vi "test All Verifies With Labels.vi"(8 "error in":errorcluster, 11 "Testing Approval Tests in":refnum<class "VITester Extension Tests.lvclass">) -> (0 "error out":errorcluster, 3 "Testing Approval Tests in":refnum<class "VITester Extension Tests.lvclass">)   [LabVIEW 2025, in "VITester Extension Tests.lvclass"]
uses:
  VITester Extension Tests.lvclass
  C:/Program Files/National Instruments/LabVIEW 2026/vi.lib/Addons/_JKI Toolkits/VI Tester/TestCase.llb/TestCase.lvclass
  Source/Approval Tests/Options/Options.lvclass/Options.ctl
  Source/Approval Tests/Naming Data/Naming Data.lvclass/Naming Data.ctl
  Caraya.Tests/Caraya Extension Tests/Utility Greet.vi
  Source/Approval Tests/Options/Options.lvclass
  Source/Approval Tests/Scrubber/Scrubber.lvclass
  Source/Approval Tests/Namer/Namer.lvclass
  Source/Approval Tests/Naming Data/Naming Data.lvclass
  Source/Approval Tests/Reporter/Reporter.lvclass
  Source/Approval Tests/Text Comparator/Text Comparator.lvclass
  VITester Extension Tests.lvclass/VITester Extension Tests.ctl
  24d0000c-8485-4d5f-9e8a-c81d323cd4a2.vi
  25835d91-223e-4457-8654-ed94975679ce.vi
  Caraya.Tests/Caraya Extension Tests/Caraya Extension Tests.lvclass
  1e735b7d-9815-499c-8608-d65425232398.vi
  Source/Extensions/VITester.Extension/VITester.Extension.lvlib
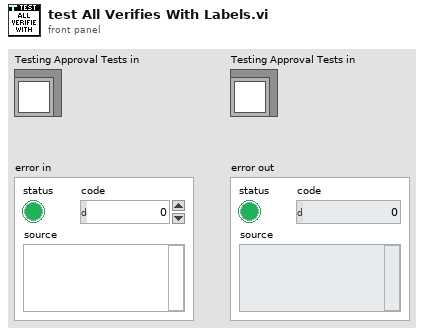
[diagram p1: front panel]
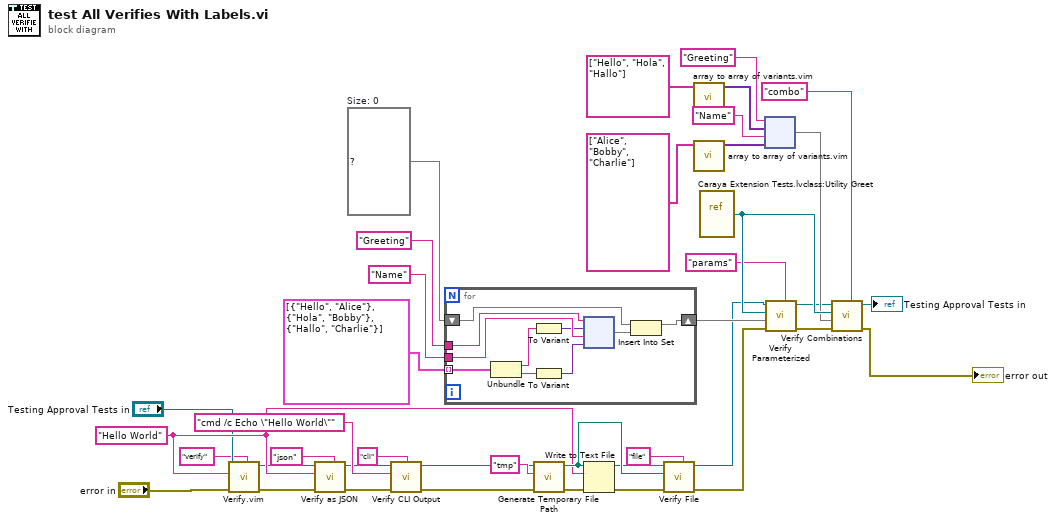
[diagram p0: block diagram]
diagram:
  w28 = set{map{string, variant}} {}  # Size: 0
  w14 = "Hello World"
  n1 = call "Verify.vim"("Label"="verify", "error in"="error in", "Test Data"=w14, "TestCase in"="Testing Approval Tests in") -> ("error out"=w39:errorcluster, "TestCase out"=w12:refnum<class "VITester Extension Tests.lvclass">)  [unwired: 6 in]
  n2 = call "Verify as JSON.vi"("Label"="json", "error in"=w39, "Anything"=w14, "TestCase in"=w12) -> ("error out"=w38:errorcluster, "TestCase out"=w11:refnum<class "VITester Extension Tests.lvclass">)  [unwired: 6 in]
  n3 = call "Verify CLI Output.vi"("Label"="cli", "error in"=w38, "command line"="cmd /c Echo \"Hello World\"", "TestCase in"=w11) -> ("error out"=w35:errorcluster, "TestCase out"=w10:refnum<class "VITester Extension Tests.lvclass">)  [unwired: 6 in]
  n4 = for {
    tunnel: "Greeting" -> [w49]
    tunnel: cluster{string, string}[] [{"Hello", "Alice"}, {"Hola", "Bobby"}, {"Hallo", "Charlie"}] -> [w47] mode=indexing
    tunnel: "Name" -> [w48]
    shift-right: [w41] -> w29
    shift-left: w28 -> [w40]
    n5 = Unbundle(w47) -> (w46:string, w45:string)
    n6 = To Variant(anything=w46) -> (Variant=w43:variant)
    n7 = To Variant(anything=w45) -> (Variant=w42:variant)
    n8 = node ("Build Map")(w49, w43, w48, w42) -> (w44:map{string, variant})
    n9 = Insert Into Set(10:w44, 11:w40) -> (3:w41:set{map{string, variant}})  [unwired: 1 out]
  }
  n10 = call <vilib>:"Generate Temporary File Path.vi"("error in (no error)"=w35, "Temporary File Extension (tmp)"="tmp") -> ("error out"=w34:errorcluster, "Unique Temporary File Path"=w15:path)  [unwired: 8 in]
  n11 = Write to Text File(file (use dialog)=w15, text=w14, error in=w34) -> (error out=w33:errorcluster)  [unwired: 1 in, 2 out]
  n12 = call "Verify File.vi"("Label"="file", "error in"=w33, "Path to Binary File to Verify"=w15, "TestCase in"=w10) -> ("error out"=w37:errorcluster, "TestCase out"=w9:refnum<class "VITester Extension Tests.lvclass">)  [unwired: 6 in]
  n13 = call "array to array of variants.vim"("Array in"=string[] ["Hello", "Hola", "Hallo"]) -> ("Array out"=w20:variant[])  [unwired: 10 in]
  n14 = call "array to array of variants.vim"("Array in"=string[] ["Alice", "Bobby", "Charlie"]) -> ("Array out"=w21:variant[])  [unwired: 10 in]
  n15 = vi-ref "Caraya Extension Tests.lvclass:Utility Greet.vi"() -> (w24:refnum<vi>)
  n16 = node ("Build Map")("Greeting" ("key"), w20, "Name" ("key"), w21) -> (w23:map{string, variant[]})
  n17 = call "Verify Parameterized.vi"("Label"="params", "error in"=w37, "Set of ctl label -> value var"=w29, "VI in"=w24, "TestCase in"=w9) -> ("error out"=w36:errorcluster, "TestCase out"=w8:refnum<class "VITester Extension Tests.lvclass">)  [unwired: 5 in]
  n18 = call "Verify Combinations.vi"("Label"="combo", "error in"=w36, "ctl label -> value var[]"=w23, "VI Refnum"=w24, "TestCase in"=w8) -> ("error out"=→"error out":errorcluster, "TestCase out"=→"Testing Approval Tests in":refnum<class "VITester Extension Tests.lvclass">)  [unwired: 5 in]
